vi "Subvi gated pixel clock generator.vi"(8 "Line clock change":bool, 9 "Pixel clock":bool, 10 "Nmax lines":u16) -> ()   [LabVIEW 2017]
uses:
  <vilib>/rvi/Emulation/niFpgaSctlEmulationGetInTimedLoop.vi
  Detector/GV start acquisition.vi
  Detector/GV gated pixel clock change.vi
  <vilib>/rvi/Emulation/niFpgaProcessEmulError.vi
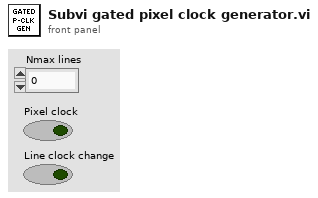
[diagram p1: front panel]
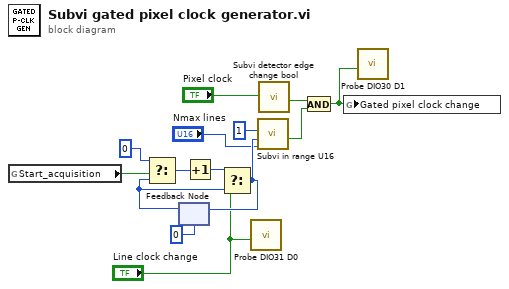
[diagram p0: block diagram]
diagram:
  n1 = global read "GV start acquisition.vi" "Start_acquisition"() -> (w3:bool)
  n2 = feedback #1(u16 0) -> (w5:u16)
  n3 = Select(t=u16 0, s=w3, f=w5) -> (s? t:f=w6:u16)
  n4 = Increment(x=w6) -> (x+1=w11:u16)
  n5 = Select(t=w11, s="Line clock change", f=w5) -> (s? t:f=w12:u16)
  n6 = feedback-in #1(w12) -> ()
  n7 = call "Probe DIO31 D0.vi"("D0"="Line clock change") -> ()  [unwired: 11 in]
  n8 = call "Subvi in range U16.vi"("Max"="Nmax lines", "Input"=w12, "Min"=u16 1) -> ("In range"=w9:bool)  [unwired: 8 in]
  n9 = call "Subvi detector edge change bool.vi"("Input"="Pixel clock") -> ("Output"=w14:bool)  [unwired: 8 in]
  n10 = And(x=w14, y=w9) -> (x .and. y?=w8:bool)
  n11 = global write "GV gated pixel clock change.vi" "Gated pixel clock change"(w8) -> ()
  n12 = call "Probe DIO30 D1.vi"("D1"=w8) -> ()  [unwired: 11 in]
